vi "configureCameras.vi"(8 "error in (no error)":errorcluster, 10 "deviceName":string, 11 "BECHWCBasic in":refnum<class "BECHWCBasic.lvclass">) -> (0 "error out":errorcluster, 3 "BECHWCBasic out":refnum<class "BECHWCBasic.lvclass">)   [LabVIEW 2011, in "Hardware.lvlib" / "HWControllers.lvlib" / "BECHWCBasic.lvclass"]
doc: "Configure this camera for the next acquisition"
uses:
  BECHWCBasic.lvclass
  BECHWCBasic.lvclass/BECHWCBasic.ctl
  Tools/Filing/FileSystem/FileSystem.lvclass
  IntegrationManagement/CameraManager.lvclass
  HWController.lvclass
  Tools/Filing.lvlib
  Tools/Filing/FileNeologist/FileNeologist.lvclass
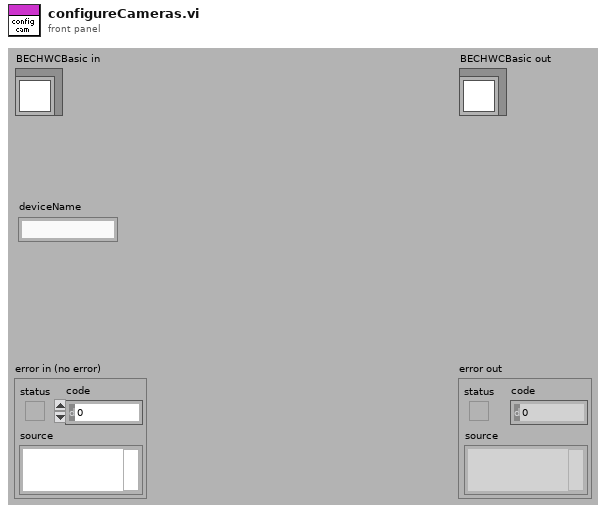
[diagram p1: front panel]
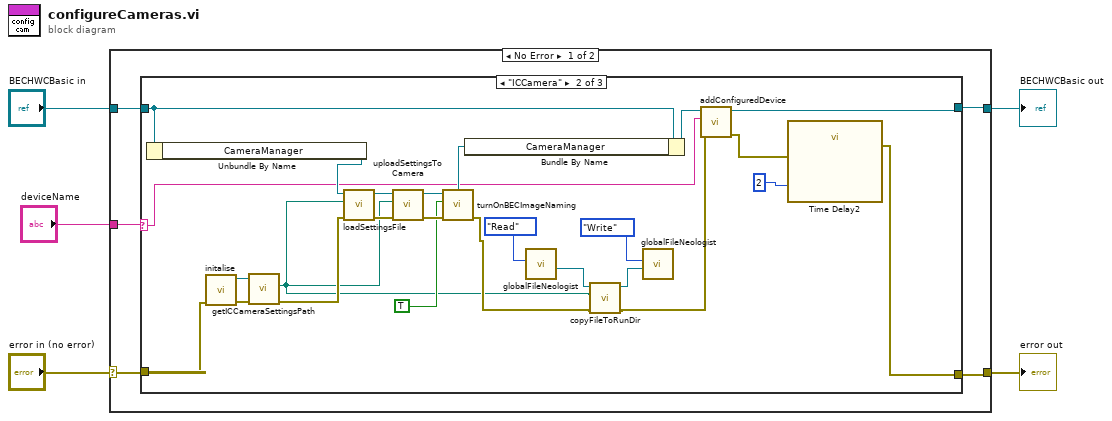
[diagram p0: block diagram]
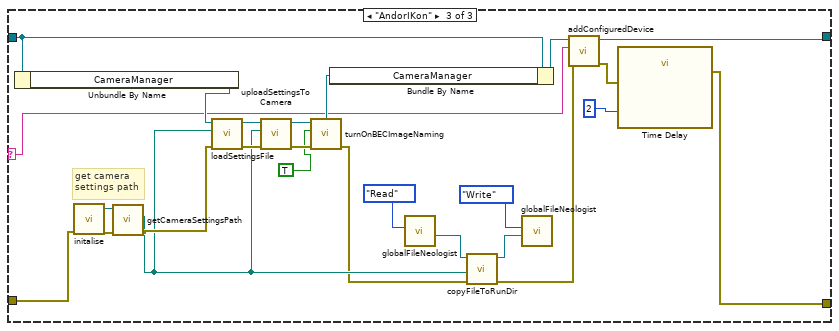
[diagram p3: hidden frame]
diagram:
  n1 = case shown="No Error" "error in (no error)" {
    selector: "error in (no error)" -> [w6 w64]
    tunnel: [w7 w64] -> w4
    tunnel: [w8 w63] -> w1
    tunnel: "BECHWCBasic in" -> [w9 w63]
    tunnel: "deviceName" -> [w10 _]
    frame No Error {
      n2 = case shown="\"ICCamera\"" w10 {
        selector: w10 -> [_ w23 w51]
        tunnel: w9 -> [w12 w37 w62]
        tunnel: [w12 w24 w52] -> w8
        tunnel: [w11 w13 w38] -> w7
        tunnel: w6 -> [w11 w31 w59]
        frame "No Hardware", Default {
        }
        frame "ICCamera" {
          n3 = Unbundle By Name(w37) -> ("CameraManager"=w34:refnum<class "CameraManager.lvclass">)
          n4 = call "initalise.vi"("error in (no error)"=w31) -> ("error out"=w36:errorcluster, "FileSystem out"=w35:refnum<class "FileSystem.lvclass">)  [unwired: 9 in]
          n5 = call-dynamic "getICCameraSettingsPath.vi"("error in (no error)"=w36, "FileSystem.lvclass in"=w35) -> ("error out"=w32:errorcluster, "ICCameraSettingsPath"=w18:path)  [unwired: 7 in, 1 out]
          n6 = call "loadSettingsFile.vi"("error in (no error)"=w32, "Path"=w18, "CameraManager in"=w34) -> ("error out"=w33:errorcluster, "CameraManager out"=w30:refnum<class "CameraManager.lvclass">)  [unwired: 7 in]
          n7 = call "uploadSettingsToCamera.vi"("error in (no error)"=w33, "Path"=w18, "CameraManager in"=w30) -> ("error out"=w28:errorcluster, "CameraManager out"=w29:refnum<class "CameraManager.lvclass">)  [unwired: 7 in]
          n8 = call "turnOnBECImageNaming.vi"("error in (no error)"=w28, "ImageRenaming"=TRUE, "CameraManager in"=w29) -> ("error out"=w20:errorcluster, "CameraManager out"=w27:refnum<class "CameraManager.lvclass">)  [unwired: 7 in]
          n9 = Bundle By Name(cluster=w37, "CameraManager"=w27) -> (w25:refnum<class "BECHWCBasic.lvclass">)
          n10 = call "globalFileNeologist.vi"("Action"=enum16{"Write", "Read"}."Read") -> ("FileNeologist out"=w17:refnum<class "FileNeologist.lvclass">)  [unwired: 10 in]
          n11 = call "copyFileToRunDir.vi"("error in (no error)"=w20, "Path"=w18, "FileNeologist in"=w17) -> ("error out"=w19:errorcluster, "FileNeologist out"=w16:refnum<class "FileNeologist.lvclass">)  [unwired: 7 in]
          n12 = call "globalFileNeologist.vi"("FileNeologist in"=w16, "Action"=enum16{"Write", "Read"}."Write") -> ()  [unwired: 9 in, 1 out]
          n13 = call "addConfiguredDevice.vi"("error in (no error)"=w19, "deviceName"=w23, "HWController in"=w25) -> ("error out"=w14:errorcluster, "HWController out"=w24:refnum<class "BECHWCBasic.lvclass">)  [unwired: 7 in]
          n14 = call "Time Delay2"("error in (no error)"=w14, "Delay Time (s)"=2) -> ("error out"=w13:errorcluster)  [unwired: 9 in]
        }
        frame "AndorIKon" {
          # "get camera\nsettings path"
          n15 = Unbundle By Name(w62) -> ("CameraManager"=w61:refnum<class "CameraManager.lvclass">)
          n16 = call "initalise.vi"("error in (no error)"=w59) -> ("error out"=w50:errorcluster, "FileSystem out"=w49:refnum<class "FileSystem.lvclass">)  [unwired: 9 in]
          n17 = call-dynamic "getCameraSettingsPath.vi"("error in (no error)"=w50, "FileSystem.lvclass in"=w49) -> ("error out"=w48:errorcluster, "CameraSettingsPath"=w47:path)  [unwired: 7 in, 1 out]
          n18 = call "loadSettingsFile.vi"("error in (no error)"=w48, "Path"=w47, "CameraManager in"=w61) -> ("error out"=w60:errorcluster, "CameraManager out"=w58:refnum<class "CameraManager.lvclass">)  [unwired: 7 in]
          n19 = call "uploadSettingsToCamera.vi"("error in (no error)"=w60, "Path"=w47, "CameraManager in"=w58) -> ("error out"=w56:errorcluster, "CameraManager out"=w57:refnum<class "CameraManager.lvclass">)  [unwired: 7 in]
          n20 = call "turnOnBECImageNaming.vi"("error in (no error)"=w56, "ImageRenaming"=TRUE, "CameraManager in"=w57) -> ("error out"=w40:errorcluster, "CameraManager out"=w55:refnum<class "CameraManager.lvclass">)  [unwired: 7 in]
          n21 = Bundle By Name(cluster=w62, "CameraManager"=w55) -> (w53:refnum<class "BECHWCBasic.lvclass">)
          n22 = call "globalFileNeologist.vi"("Action"=enum16{"Write", "Read"}."Read") -> ("FileNeologist out"=w42:refnum<class "FileNeologist.lvclass">)  [unwired: 10 in]
          n23 = call "copyFileToRunDir.vi"("error in (no error)"=w40, "Path"=w47, "FileNeologist in"=w42) -> ("error out"=w39:errorcluster, "FileNeologist out"=w41:refnum<class "FileNeologist.lvclass">)  [unwired: 7 in]
          n24 = call "globalFileNeologist.vi"("FileNeologist in"=w41, "Action"=enum16{"Write", "Read"}."Write") -> ()  [unwired: 9 in, 1 out]
          n25 = call "addConfiguredDevice.vi"("error in (no error)"=w39, "deviceName"=w51, "HWController in"=w53) -> ("error out"=w46:errorcluster, "HWController out"=w52:refnum<class "BECHWCBasic.lvclass">)  [unwired: 7 in]
          n26 = call "Time Delay"("error in (no error)"=w46, "Delay Time (s)"=2) -> ("error out"=w38:errorcluster)  [unwired: 9 in]
        }
      }
    }
    frame Error {
    }
  }
  "error out" <- w4
  "BECHWCBasic out" <- w1
